vi "Actor Core.vi"(8 "error in":errorcluster, 11 "Caller B in":refnum<class "Caller A.lvclass">) -> (0 "error out":errorcluster, 3 "Actor out":refnum<class "Actor.lvclass">)   [LabVIEW 2023, in "Caller A.lvlib" / "Caller A.lvclass"]
doc: "(<B>Filename</B>: Actor Framework.lvlib:Actor.lvclass:Actor Core.vi)\n\nReceives messages to the actor, reacts to them, and initiates any error handling that may shut the actor down.\n\nDescendant classes may override this VI to append parallel tasks for the actor to complete while it handles messages. Overrides use the Call Parent Method node."
uses:
  Caller A.lvclass
  c:/dev/_r/4/eng/lv-core/lvpostprocessingd/lv_mc_x86_64/dist_i386/vi.lib/ActorFramework/Actor/Actor.lvclass
  <vilib>/ActorFramework/Actor/Actor.lvclass
  Nested/Nested/Nested.lvclass
  <vilib>/ActorFramework/Actor/Actor.lvclass/Actor.ctl
  <vilib>/ActorFramework/Message Enqueuer/Message Enqueuer.lvclass/Message Enqueuer.ctl
  Caller A.lvclass/Caller A.ctl
  Nested/Nested/Named Value.ctl
  Nested/Nested Messages/Lookup Value Msg/Lookup Value Msg.lvclass/Lookup Value Msg.ctl
  <vilib>/ActorFramework/Message Enqueuer/Init from Existing Queue.vi
  <vilib>/ActorFramework/Message Enqueuer/Enqueue.vi
  <vilib>/ActorFramework/Stop Msg/Stop Msg.lvclass
  c:/dev/_r/4/eng/lv-core/lvpostprocessingd/lv_mc_x86_64/dist_i386/vi.lib/ActorFramework/Message/Message.lvclass
  Nested/Nested Messages/Lookup Value Msg/Lookup Value Msg.lvclass
  <vilib>/ActorFramework/Message Priority Queue/Priority Enqueue.vi
  <vilib>/ActorFramework/Message Enqueuer/Message Enqueuer.lvclass
panel:
  out "Meter":dbl(knob) scale=0.0..5.0
  in  "stop":bool
  in  "lookup golden ratio":bool
  in  "lookup e":bool
  in  "lookup pi":bool
  # "A"
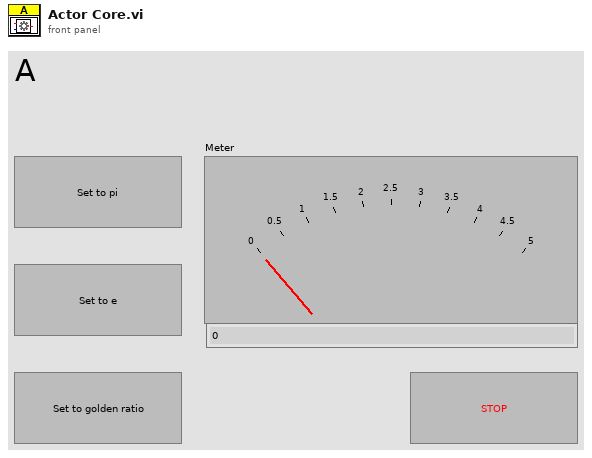
[diagram p1: front panel]
types:
  T1 = typedef "Nested.lvlib/Nested.lvclass/Named Value.ctl" = enum16{"e", "pi", "golden ratio"}
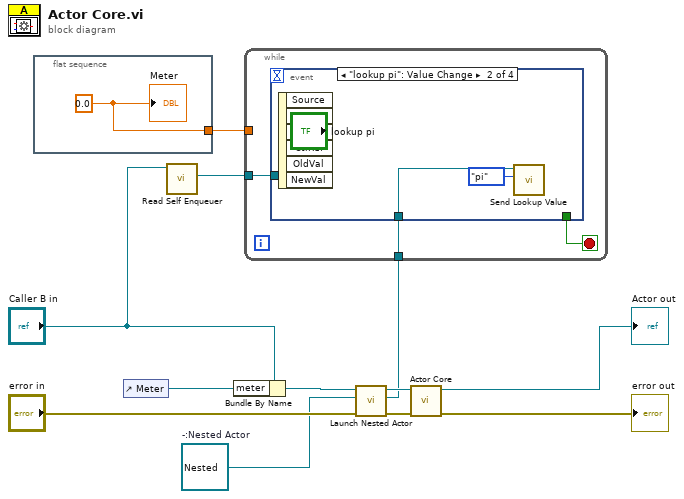
[diagram p0: block diagram]
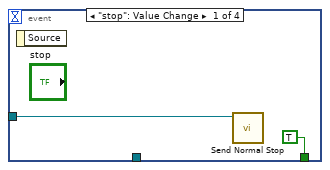
[diagram p2: hidden frame]
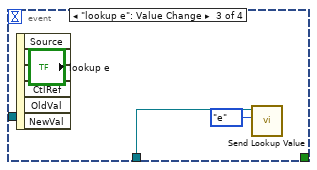
[diagram p3: hidden frame]
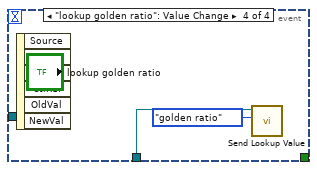
[diagram p4: hidden frame]
diagram:
  w7 = refnum<class "Nested.lvclass"> refnum  # -:Nested Actor
  n1 = flat-sequence {
    tunnel: [w13] -> w2
    frame #0 {
      w13 = 0.0 ("Meter")
      "Meter" <- w13
    }
  }
  n2 = control-ref of="Meter"() -> (w1:refnum<vi>)
  n3 = call <vilib>:"Read Self Enqueuer.vi"("Actor"="Caller B in") -> ("Self Enqueuer"=w4:refnum<class "Message Enqueuer.lvclass">)  [unwired: 10 in]
  n4 = Bundle By Name(cluster="Caller B in", "meter"=w1) -> (w6:refnum<class "Caller A.lvclass">)
  n5 = call <vilib>:"Launch Nested Actor.vi"("error in (no error)"="error in", "Nested Actor"=w7, "Caller Actor in"=w6) -> ("error out"=w9:errorcluster, "Nested Actor's Enqueuer"=w3:refnum<class "Message Enqueuer.lvclass">, "Caller Actor out"=w10:refnum<class "Caller A.lvclass">)  [unwired: 6 in]
  n6 = while {
    tunnel: w4 -> [w15]
    tunnel: w3 -> [w14]
    tunnel: w2 -> [_]
    stop <- w16 stop-if-true
    n7 = event shown="[1] \"lookup pi\": Value Change" {
      selector: _ -> [_ _ _ _]
      dyn-events: _ -> [_ _ _ _]
      timeout: _ -> [_ _ _ _]
      tunnel: [TRUE _ _ _] -> w16
      tunnel: w15 -> [w17 _ _ _]
      tunnel: w14 -> [_ w20 w22 w24]
      event "stop": Value Change {
        n8 = event-data() -> ()  [unwired: 1 in, 1 out]
        n9 = call <vilib>:"Send Normal Stop.vi"("Message Enqueuer"=w17) -> ()  [unwired: 10 in, 1 out]
      }
      event "lookup pi": Value Change {
        n10 = event-data() -> ()  [unwired: 1 in, 6 out]
        n11 = call "Send Lookup Value.vi"("named value"=Named_Value."pi", "Message Enqueuer"=w20) -> ()  [unwired: 8 in, 2 out]
      }
      event "lookup e": Value Change {
        n12 = event-data() -> ()  [unwired: 1 in, 6 out]
        n13 = call "Send Lookup Value.vi"("named value"=Named_Value."e", "Message Enqueuer"=w22) -> ()  [unwired: 8 in, 2 out]
      }
      event "lookup golden ratio": Value Change {
        n14 = event-data() -> ()  [unwired: 1 in, 6 out]
        n15 = call "Send Lookup Value.vi"("named value"=Named_Value."golden ratio", "Message Enqueuer"=w24) -> ()  [unwired: 8 in, 2 out]
      }
    }
  }
  n16 = call-parent "Actor Core.vi"("error in"=w9, "Actor in"=w10) -> ("error out"=→"error out":errorcluster, "Actor out"=→"Actor out":refnum<class "Actor.lvclass">)  [unwired: 8 in]
